vi "Witness INIT.vi"(0 "address string":string) -> ()   [LabVIEW 2010]
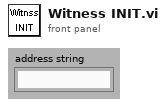
[diagram p1: front panel]
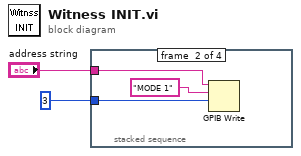
[diagram p0: block diagram]
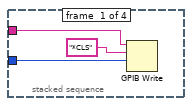
[diagram p2: hidden frame]
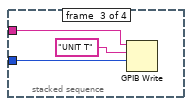
[diagram p3: hidden frame]
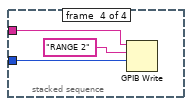
[diagram p4: hidden frame]
diagram:
  n1 = stacked-sequence {
    tunnel: "address string" -> [w4 w7 w10 w13]
    tunnel: i16 3 ("mode (0)") -> [w5 w8 w11 w14]
    frame #0 {
      n2 = GPIB Write(0:w4, 1:"*CLS" ("data"), 2:w5) -> ()  [unwired: 2 in, 2 out]
    }
    frame #1 {
      n3 = GPIB Write(0:w7, 1:"MODE 1" ("data"), 2:w8) -> ()  [unwired: 2 in, 2 out]
    }
    frame #2 {
      n4 = GPIB Write(0:w10, 1:"UNIT T" ("data"), 2:w11) -> ()  [unwired: 2 in, 2 out]
    }
    frame #3 {
      n5 = GPIB Write(0:w13, 1:"RANGE 2" ("data"), 2:w14) -> ()  [unwired: 2 in, 2 out]
    }
  }
